vi "Configure Multi Eval Meas List Segment Range.vi"(7 "Segments (10)":i32=10, 8 "error in (no error)":errorcluster, 9 "Start Index (1)":i32=1, 10 "Instance (1)":T1=1, 11 "VISA resource name":refnum<visa-resource-name>) -> (0 "error out":errorcluster, 3 "VISA resource name out":refnum<visa-resource-name>)   [LabVIEW 2020, in "Rohde&Schwarz CMWXP NR FR1 Measurement.lvlib"]
doc: "Select a range of measured segments.\n\nAttribute:\nRSCMWXPNRFR1M_ATTR_MULTI_EVAL_MEAS_LIST_SEGMENT_RANGE\n\nRemote-control command:\nCONFigure:NRSub:MEAS<i>:MEValuation:LIST:LRANge"
uses:
  <instrlib>/Rohde&Schwarz CMWXP NR FR1 Measurement/Rohde&Schwarz CMWXP NR FR1 Measurement.lvlib
  <instrlib>/Rohde&Schwarz CMWXP NR FR1 Measurement/Private/_Instance.ctl
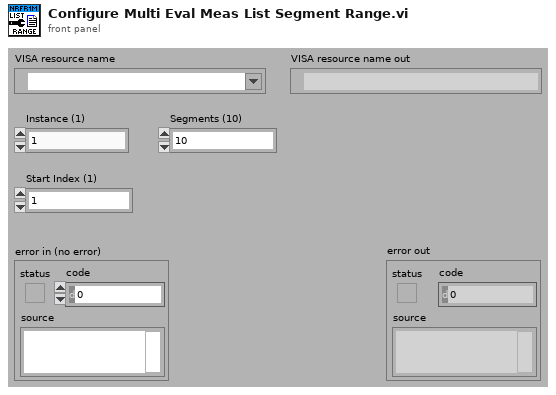
[diagram p1: front panel]
types:
  T1 = typedef "Rohde&Schwarz CMWXP NR FR1 Measurement.lvlib/_Instance.ctl" = i32
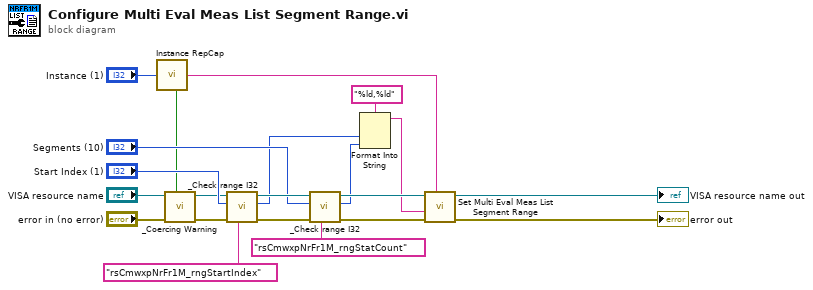
[diagram p0: block diagram]
diagram:
  n1 = call <instrlib>:"Instance RepCap.vi"("Instance In"="Instance (1)") -> ("In Range?"=w1:bool, "RepCap Identifier Out"=w18:string)  [unwired: 1 in]
  n2 = call <instrlib>:"_Coercing Warning.vi"("In Range?"=w1, "error in (no error)"="error in (no error)", "VISA resource name"="VISA resource name") -> ("error out"=w3:errorcluster, "VISA resource name out"=w2:refnum<visa-resource-name>)  [unwired: 7 in]
  n3 = call <instrlib>:"_Check range I32.vi"("Range Table Identifier"="rsCmwxpNrFr1M_rngStartIndex", "error in (no error)"=w3, "I32 Value In"="Start Index (1)", "VISA resource name"=w2) -> ("error out"=w17:errorcluster, "I32 Value Out"=w9:i32, "VISA resource name out"=w16:refnum<visa-resource-name>)  [unwired: 5 in]
  n4 = call <instrlib>:"_Check range I32.vi"("Range Table Identifier"="rsCmwxpNrFr1M_rngStatCount", "error in (no error)"=w17, "I32 Value In"="Segments (10)", "VISA resource name"=w16) -> ("error out"=w15:errorcluster, "I32 Value Out"=w7:i32, "VISA resource name out"=w14:refnum<visa-resource-name>)  [unwired: 5 in]
  n5 = Format Into String(format string="%ld,%ld", w9, w7) -> (resulting string=w6:string)  [unwired: 2 in, 1 out]
  n6 = call "Set Multi Eval Meas List Segment Range"("Repeated Capabilities"=w18, "error in (no error)"=w15, "Multi Eval Meas List Segment Range ()"=w6, "instrument handle"=w14) -> ("error out"=→"error out":errorcluster, "instrument handle out"=→"VISA resource name out":refnum<visa-resource-name>)  [unwired: 6 in]
